vi "SimpleExample Synchronous Query.vi"() -> ()   [LabVIEW 2011]
uses:
  Interprocess Messenger/QueueMessenger/QueueMessenger.lvclass
  Interprocess Messenger/TextVarientMessage/MSG.lvclass
  Interprocess Messenger/Send/Send.lvclass
  Interprocess Messenger/Send/Send (no data).vi
  Interprocess Messenger/Send/Query (varients).vi
  Interprocess Messenger/TextVarientMessage/Reply (varient).vi
panel:
  out "Time":timestamp
  # "Any Key Down to stop"
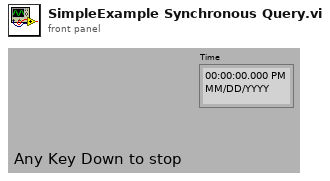
[diagram p1: front panel]
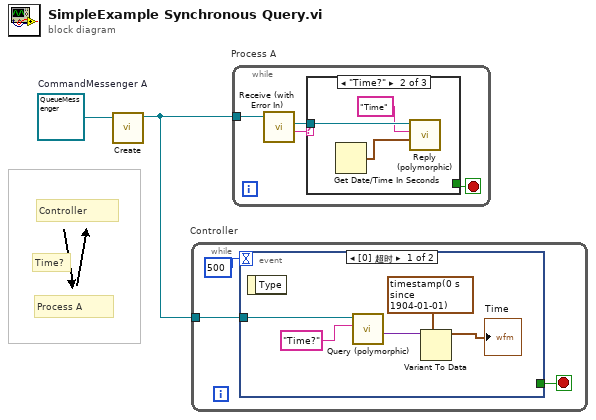
[diagram p0: block diagram]
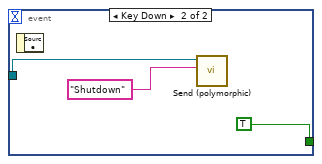
[diagram p2: hidden frame]
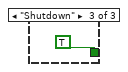
[diagram p4: hidden frame]
diagram:
  w2 = refnum<class "QueueMessenger.lvclass"> refnum  # CommandMessenger A
  # "Time?"
  # "Process A"
  # "Controller"
  n1 = call-dynamic "Create.vi"("QueueMessenger in"=w2) -> ("QueueMessenger out"=w1:refnum<class "QueueMessenger.lvclass">)  [unwired: 1 in, 9 out]
  n2 = while "Controller" {
    tunnel: w1 -> [w5]
    stop <- w4 stop-if-true
    n3 = event shown="[0] 超时" {
      selector: _ -> [_ _]
      dyn-events: _ -> [_ _]
      timeout: 500 -> [_ _]
      tunnel: w5 -> [w10 w12]
      tunnel: [_ TRUE] -> w4
      event Timeout {
        n4 = event-data() -> ()  [unwired: 2 out]
        n5 = call-poly "Query (polymorphic).vi"("Label"="Time?", "MSR Parent"=w10) -> ("Replay Varient"=w8:variant)  [unwired: 2 in, 7 out]
        n6 = Variant To Data(type=timestamp(0 s since 1904-01-01) ("current time"), Variant=w8) -> (data=→"Time":timestamp)  [unwired: 1 in, 1 out]
      }
      event Key Down {
        n7 = event-data() -> ()  [unwired: 2 out]
        n8 = call-poly "Send (polymorphic).vi"("Label"="Shutdown", "MSR Parent in"=w12) -> ()  [unwired: 1 in, 9 out]
      }
    }
  }
  n9 = while "Process A" {
    tunnel: w1 -> [w17]
    stop <- w14 stop-if-true
    n10 = call-dynamic "Receive (with Error In).vi"("MGR in"=w17) -> ("Label"=w16:string, "Message"=w15:refnum<class "MSG.lvclass">)  [unwired: 2 in, 7 out]
    n11 = case shown="\"Time?\"" w16 {
      tunnel: w15 -> [_ w20 _]
      tunnel: [_ _ TRUE] -> w14
      frame "False", Default {
      }
      frame "Time?" {
        n12 = Get Date/Time In Seconds() -> (seconds since 1Jan1904=w19:timestamp)
        n13 = call-poly "Reply (polymorphic).vi"("Varient"=w19, "Reply"="Time", "Message to Reply to"=w20) -> ()  [unwired: 1 in, 8 out]
      }
      frame "Shutdown" {
      }
    }
  }
